vi "Add Index (Dnet CommandRegister Buffer).vi"(8 "Count":i32, 10 "Value":bool, 11 "Indices Input":i32[](array[numeric])) -> (0 "Count+1":i32, 3 "Indices Output":i32[](array[numeric]))   [LabVIEW 2011]
uses:
  GlobalVariables.vi
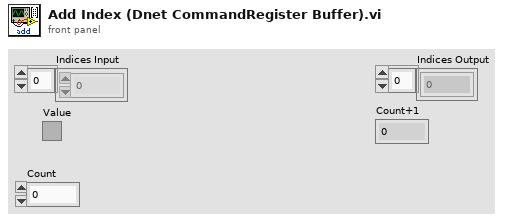
[diagram p1: front panel]
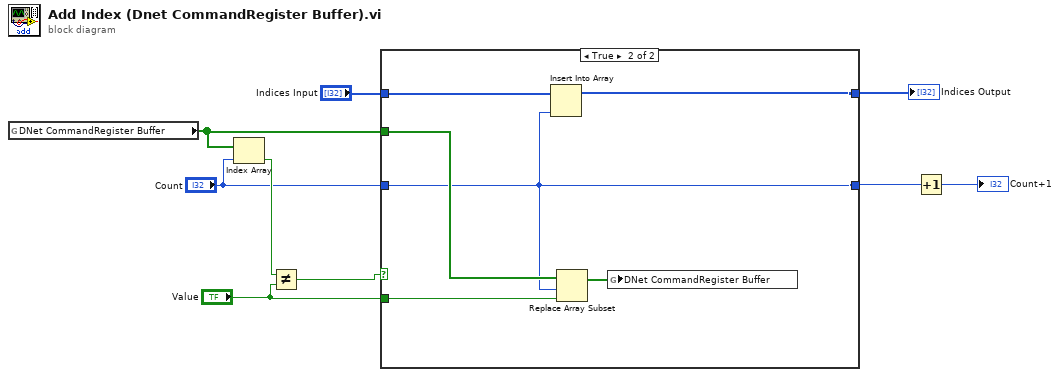
[diagram p0: block diagram]
diagram:
  n1 = global read "GlobalVariables.vi" "DNet CommandRegister Buffer"() -> (w9:bool[])
  n2 = Index Array(array=w9, index="Count") -> (element=w8:bool)
  n3 = Not Equal?(x=w8, y="Value") -> (x != y?=w1:bool)
  n4 = case shown="True" w1 {
    tunnel: w9 -> [_ w16]
    tunnel: "Indices Input" -> [w11 w15]
    tunnel: [w11 w14] -> w6
    tunnel: "Value" -> [_ w13]
    tunnel: "Count" -> [w10 w12]
    tunnel: [w10 w12] -> w3
    frame False {
    }
    frame True {
      n5 = Insert Into Array(array=w15, new element=w12) -> (w14:i32[])  [unwired: 1 in]
      n6 = Replace Array Subset(array=w16, new element=w13, index=w12) -> (w17:bool[])
      n7 = global write "GlobalVariables.vi" "DNet CommandRegister Buffer"(w17) -> ()
    }
  }
  "Indices Output" <- w6
  n8 = Increment(x=w3) -> (x+1=→"Count+1":i32)
